vi "pb-program.vi"(10 "Commands":T1(array[cluster]) {"Time" format="%.3p"; "Op Code" items=["Continue", "Stop", "Loop", "End Loop", "JSR", "RTS", "Branch", "Long Delay", "Wait"]}) -> (3 "path out":path)   [LabVIEW 2018]
panel:
  # "1"
  # "2"
  # "3"
  # "4"
  # "5"
  # "6"
  # "7"
  # "8"
  # "9"
  # "10"
  # "11"
  # "12"
  # "13"
  # "14"
  # "15"
  # "16"
  # "17"
  # "18"
  # "19"
  # "20"
  # "21"
  # "22"
  # "23"
  # "24"
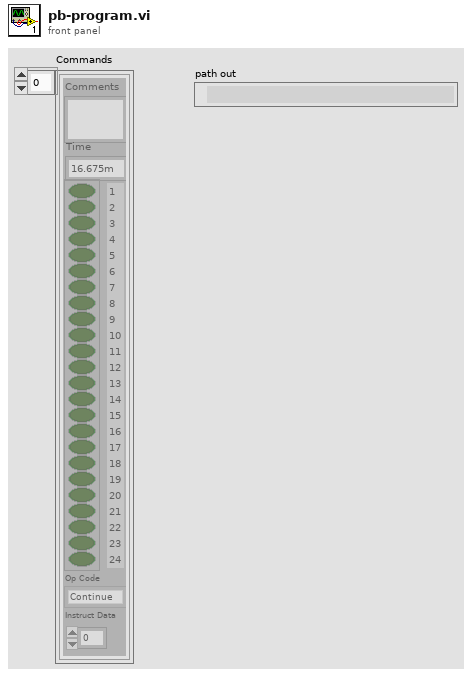
[diagram p1: front panel]
types:
  T1 = cluster{"Instruct Data":i32, "Op Code":i32, "Flags":bool[], "Comments":string, "Time":dbl}[]
  T2 = enum16{"Pulse Program", "Frequency Registers", "TX Phase Registers", "RX Phase Registers"}
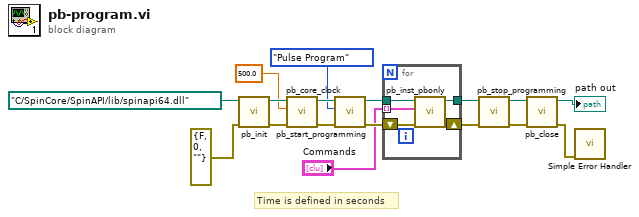
[diagram p0: block diagram]
diagram:
  # "Time is defined in seconds"
  n1 = call "pb_init.vi"("error in (no error)"=errorcluster {"status"=FALSE, "code"=0, "source"=""} ("error constant"), "path in"=path "C:/SpinCore/SpinAPI/lib/spinapi64.dll") -> ("error out"=w15:errorcluster, "path out"=w16:path)  [unwired: 8 in]
  n2 = call "pb_core_clock.vi"("error in (no error)"=w15, "clock_freq (MHz)"=500.0, "path in"=w16) -> ("error out"=w12:errorcluster, "path out"=w13:path)  [unwired: 7 in]
  n3 = call "pb_start_programming.vi"("error in (no error)"=w12, "Device"=T2."Pulse Program", "path in"=w13) -> ("error out"=w7:errorcluster, "path out"=w8:path)  [unwired: 7 in]
  n4 = for {
    tunnel: "Commands" -> [w22] mode=indexing
    tunnel: [w21] -> w6
    tunnel: w8 -> [w20]
    shift-right: [w18] -> w5
    shift-left: w7 -> [w19]
    n5 = call "pb_inst_pbonly.vi"("error in (no error)"=w19, "PB Instruction"=w22, "path in"=w20) -> ("error out"=w18:errorcluster, "path out"=w21:path)  [unwired: 7 in]
  }
  n6 = call "pb_stop_programming.vi"("error in (no error)"=w5, "path in"=w6) -> ("error out"=w9:errorcluster, "path out"=w10:path)  [unwired: 8 in]
  n7 = call "pb_close.vi"("error in (no error)"=w9, "path in"=w10) -> ("error out"=w1:errorcluster, "path out"=→"path out":path)  [unwired: 8 in]
  n8 = call <vilib>:"Simple Error Handler.vi"("error in (no error)"=w1) -> ()  [unwired: 4 in, 5 out]
